vi "Perform Step.vi"(8 "error in (no error)":errorcluster, 11 "Keyboard Action in":refnum<class "Keyboard Action.lvclass">) -> (0 "error out":errorcluster, 2 "Result":T1, 3 "Keyboard Action out":refnum<class "Keyboard Action.lvclass">)   [LabVIEW 2020, in "MacroAssert.lvlib" / "Keyboard Action.lvclass"]
uses:
  Keyboard Action.lvclass
  C:/Users/acasalen/Documents/LabVIEW Data/Projects/MacroAssert/source/Classes/Step/Step.lvclass
  CTLs/Report Data.ctl
  MacroAssert.lvlib
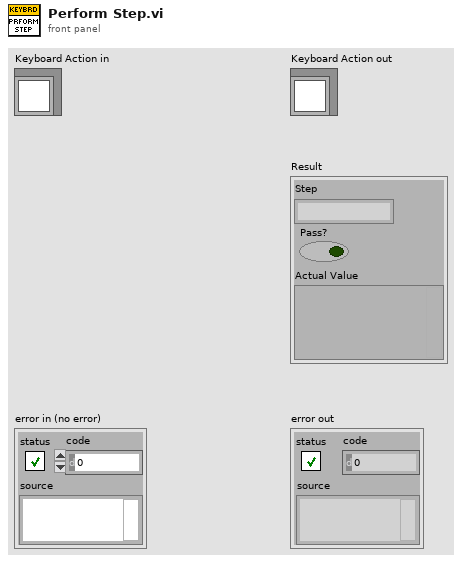
[diagram p1: front panel]
types:
  T1 = typedef "MacroAssert.lvlib/Report Data.ctl" = cluster{"Step":string, "Pass?":bool, "Actual Value":variant}
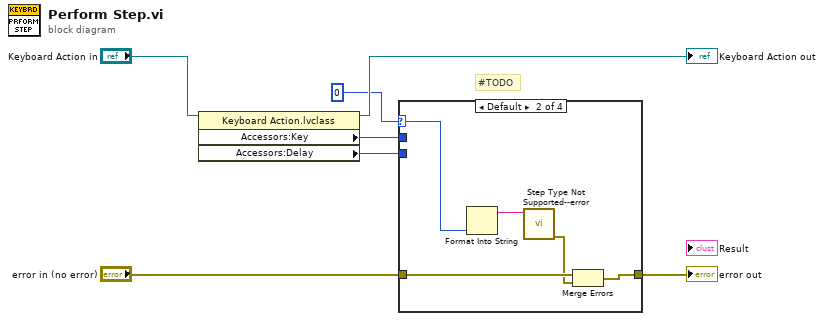
[diagram p0: block diagram]
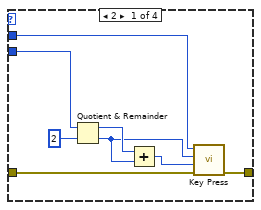
[diagram p2: hidden frame]
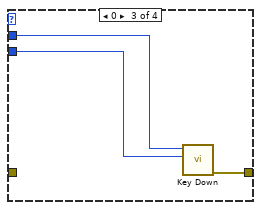
[diagram p3: hidden frame]
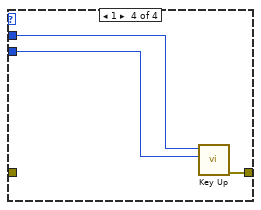
[diagram p4: hidden frame]
diagram:
  # "#TODO"
  n1 = property class="Keyboard Action.lvclass"(reference="Keyboard Action in") -> (reference out=→"Keyboard Action out":refnum<class "Keyboard Action.lvclass">, "Accessors:Key"=w3:u8, "Accessors:Delay"=w2:i32)  [unwired: 1 in, 1 out]
  n2 = case shown="Default" 0 {
    selector: 0 -> [_ w20 _ _]
    tunnel: w2 -> [w14 _ w22 w25]
    tunnel: w3 -> [w9 _ w21 w24]
    tunnel: [w15 w16 w23 w26] -> w4
    tunnel: "error in (no error)" -> [w8 w18 _ _]
    frame 2 {
      n3 = Quotient & Remainder(x=w14, y=2) -> (x-y*floor(x/y)=w12:i32, floor(x/y)=w10:i32)
      n4 = Add(x=w12, y=w10) -> (x+y=w11:i32)
      n5 = call "Key Press.vi"("error in (no error)"=w8, "ms wait after up (20)"=w11, "ms wait after down (80)"=w10, "Virtual Key"=w9) -> ("error out"=w15:errorcluster)  [unwired: 7 in]
    }
    frame Default {
      n6 = Format Into String(w20) -> (resulting string=w19:string)  [unwired: 3 in, 1 out]
      n7 = call "Step Type Not Supported--error.vi"("Step Type"=w19) -> ("error out"=w17:errorcluster)  [unwired: 10 in]
      n8 = Merge Errors(w18, w17) -> (w16:errorcluster)
    }
    frame 0 {
      n9 = call "Key Down.vi"("delay in ms (80)"=w22, "Virtual Key"=w21) -> ("error out"=w23:errorcluster)  [unwired: 9 in]
    }
    frame 1 {
      n10 = call "Key Up.vi"("delay in ms (20)"=w25, "Virtual Key"=w24) -> ("error out"=w26:errorcluster)  [unwired: 9 in]
    }
  }
  "error out" <- w4
